vi "CRYCheck TS Existing.vi"(11 "Sequence Name In":string) -> (2 "Is Read?":bool, 3 "Is Replace?":bool)   [LabVIEW 2013]
uses:
  CRYProject Editor Global.vi
  CRYSystem/Calibration/SubVI/CRYCal Global.vi
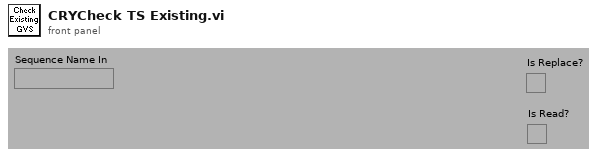
[diagram p1: front panel]
types:
  T1 = typedef "CRYTS.ctl" = cluster{"No.TS":u16, "TS File Path":path, "TS Name":string, "EditStepName":string, "Steps":T2[], "New State":bool, "Change State":bool, "Flattened CurveLib Data":string, "Document Data":string, "EditStepNo":u16, "Operator Start File":string, "Sequence Type":string, "Sequence Language":string}
  T2 = typedef "CRYStep.ctl" = cluster{"No.VI":i32, "Category":string, "StepName":string, "Seq setup flattened":string, "Comment":string, "Steps config.":bool[], "Jump config":i32[], "Start":dbl, "Increment":dbl, "Name":string, "Unit":string, "Y data":u16, "Y prefix":string, "Y dB ref":dbl, "Y unit":string, "Repeat State Array":cluster{"Start":dbl, "Increment":dbl, "Count":i32, "Num":i32}[]}
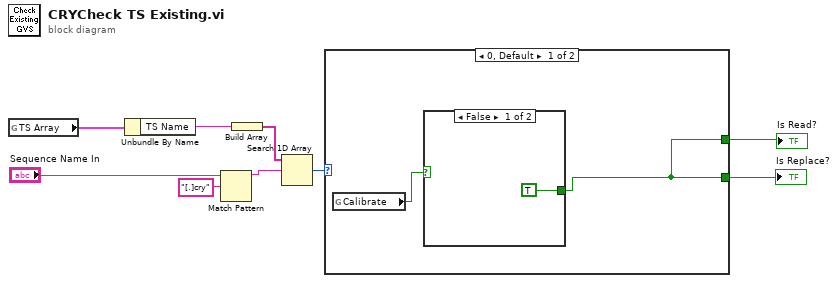
[diagram p0: block diagram]
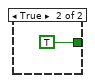
[diagram p2: hidden frame]
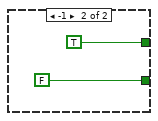
[diagram p3: hidden frame]
diagram:
  n1 = global read "CRYProject Editor Global.vi" "TS Array"() -> (w6:T1)
  n2 = Unbundle By Name(w6) -> ("TS Name"=w8:string)
  n3 = Match Pattern(string="Sequence Name In", regular expression="[.]cry") -> (before substring=w7:string)  [unwired: 4 out]
  n4 = Build Array(w8) -> (w1:string[])
  n5 = Search 1D Array(1D array=w1, element=w7) -> (index of element=w4:i32)  [unwired: 1 out]
  n6 = case shown="0, Default" w4 {
    tunnel: [w10 FALSE ("Is Replace?")] -> w3
    tunnel: [w10 TRUE ("f")] -> w2
    frame 0, Default {
      n7 = global read "CRYCal Global.vi" "Calibrate"() -> (w11:bool)
      n8 = case shown="False" w11 {
        tunnel: [TRUE ("Is Replace?") TRUE ("T button?")] -> w10
        frame False {
        }
        frame True {
        }
      }
    }
    frame -1 {
    }
  }
  "Is Replace?" <- w3
  "Is Read?" <- w2
